vi "Create Initialize VIs.vi"   [LabVIEW 2015]
uses:
  Project Manipulation Scripts/Project Manipulation Scripts.lvlib
types:
  T1 = enum32{"invalid scope", "public", "private", "protected", "community"}
  T2 = enum32{"Invalid", "Standard", "Closed", "Hidden", "Minimized", "Maximized"}
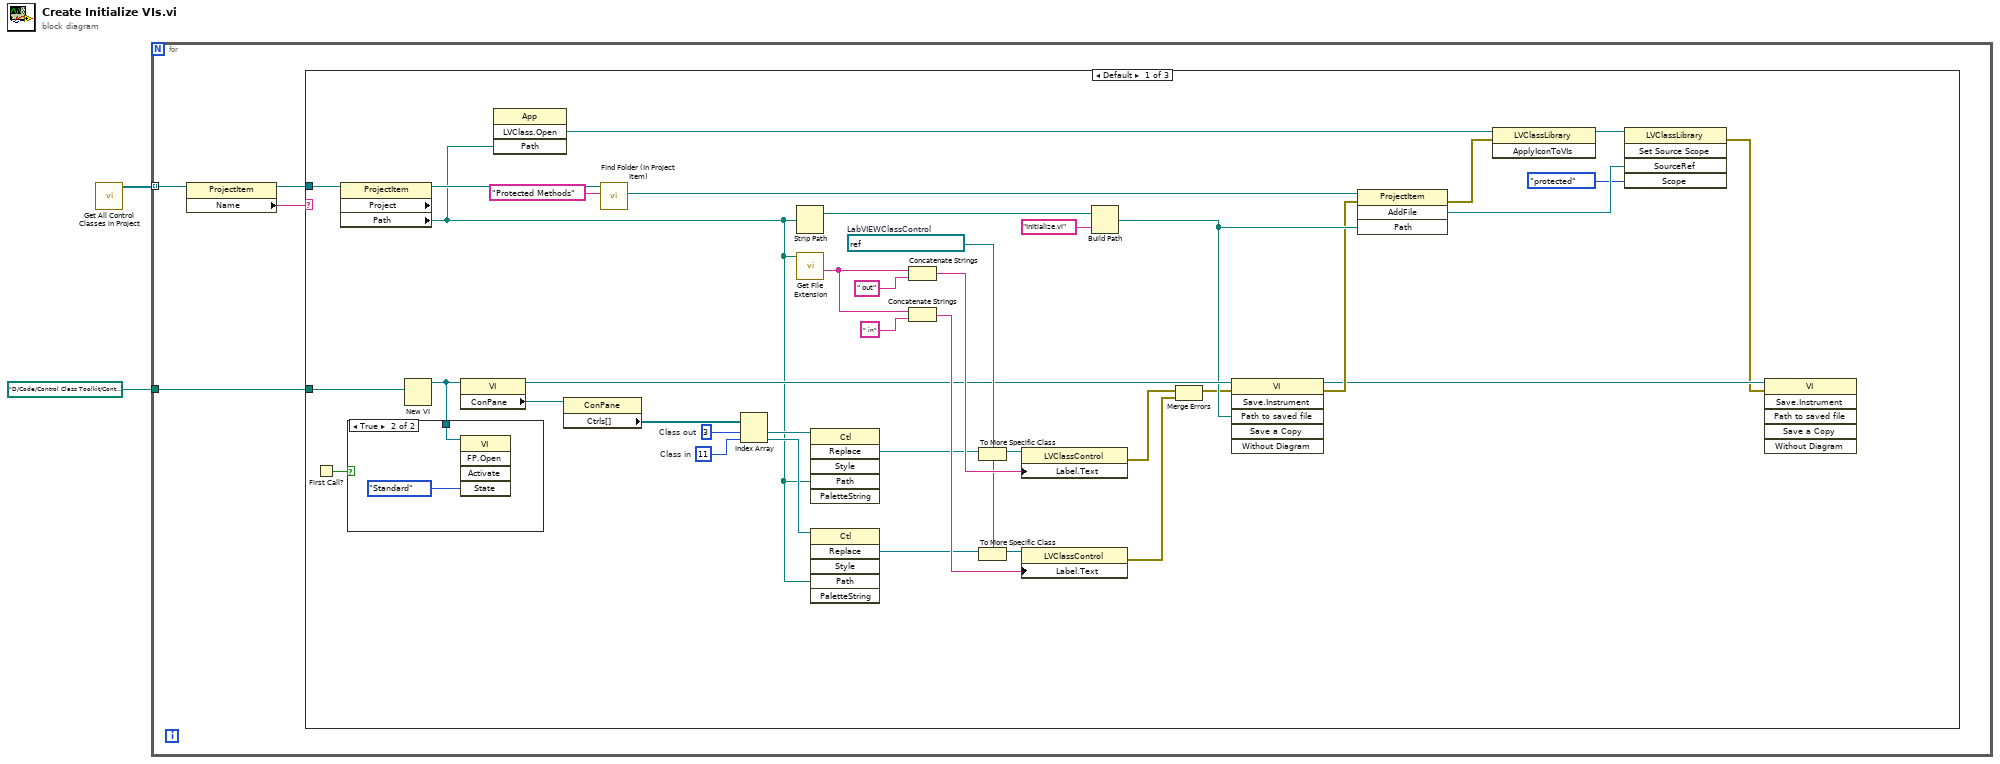
[diagram p0: block diagram]
diagram:
  n1 = call "Get All Control Classes in Project.vi"() -> ("All Control Classes"=w2:refnum<vi>[])  [unwired: 11 in]
  n2 = for {
    tunnel: w2 -> [w6] mode=indexing
    tunnel: path "D:/Code/Control Class Toolkit/Control Classes/Array/Initialize.vi" -> [w3]
    n3 = property class="ProjectItem"(reference=w6) -> (reference out=w4:refnum<vi>, "Name"=w5:string)  [unwired: 1 in, 1 out]
    n4 = case shown="Default" w5 {
      tunnel: w4 -> [w45 _ _]
      tunnel: w3 -> [w44 _ _]
      frame Default {
        w27 = refnum<vi> refnum  # LabVIEWClassControl
        w40 = 11  # Class in
        w41 = 3  # Class out
        n5 = First Call?() -> (First Call?: T/F=w7:bool)
        n6 = property class="ProjectItem" props=["Project", "Path"](reference=w45) -> (reference out=w22:refnum<vi>, "Path"=w15:path)  [unwired: 1 in, 2 out]
        n7 = New VI(10:w44) -> (3:w37:refnum<vi>)  [unwired: 6 in, 1 out]
        n8 = case shown="True" w7 {
          tunnel: w37 -> [_ w47]
          frame False {
          }
          frame True {
            n9 = invoke class="VI" method="FP.Open"(reference=w47, "State"=T2."Standard") -> ()  [unwired: 3 in, 5 out]
          }
        }
        n10 = property class="VI"(reference=w37) -> (reference out=w24:refnum<vi>, "ConPane"=w43:refnum<vi>)  [unwired: 1 in, 1 out]
        n11 = invoke class="App" method="LVClass.Open"("Path"=w15) -> ("LVClass.Open"=w14:refnum<vi>)  [unwired: 3 in, 3 out]
        n12 = property class="ConPane"(reference=w43) -> ("Ctrls[]"=w42:refnum<vi>[])  [unwired: 1 in, 2 out]
        n13 = call "Find Folder (In Project Item).vi"("Folder Name"="Protected Methods", "ProjectItem in"=w22) -> ("Folder Refnum"=w21:refnum<vi>)  [unwired: 7 in, 2 out]
        n14 = Index Array(array=w42, index #1=w41, index #2=w40) -> (element #1=w39:refnum<vi>, element #2=w38:refnum<vi>)
        n15 = Strip Path(path=w15) -> (stripped path=w26:path)  [unwired: 1 out]
        n16 = call <vilib>:"Get File Extension.vi"("file"=w15) -> ("filename without extension"=w34:string)  [unwired: 6 in, 4 out]
        n17 = invoke class="Ctl" method="Replace"(reference=w39, "Path"=w15) -> ("Replace"=w31:refnum<vi>)  [unwired: 4 in, 5 out]
        n18 = invoke class="Ctl" method="Replace"(reference=w38, "Path"=w15) -> ("Replace"=w29:refnum<vi>)  [unwired: 4 in, 5 out]
        n19 = Concatenate Strings(w34, " out" ("Label.Text")) -> (w33:string)
        n20 = Concatenate Strings(w34, " in" ("Label.Text")) -> (w32:string)
        n21 = To More Specific Class(target class=w27, reference=w31) -> (specific class reference=w30:refnum<vi>)  [unwired: 1 in, 1 out]
        n22 = To More Specific Class(target class=w27, reference=w29) -> (specific class reference=w28:refnum<vi>)  [unwired: 1 in, 1 out]
        n23 = property class="LVClassControl"(reference=w30, "Label.Text"=w33) -> (error out=w18:errorcluster)  [unwired: 1 in, 1 out]
        n24 = property class="LVClassControl"(reference=w28, "Label.Text"=w32) -> (error out=w17:errorcluster)  [unwired: 1 in, 1 out]
        n25 = Build Path(base path=w26, name or relative path="Initialize.vi") -> (appended path=w23:path)
        n26 = Merge Errors(w18, w17) -> (w16:errorcluster)
        n27 = invoke class="VI" method="Save.Instrument"(reference=w24, error in=w16, "Path to saved file"=w23) -> (reference out=w12:refnum<vi>, error out=w19:errorcluster)  [unwired: 3 in, 4 out]
        n28 = invoke class="ProjectItem" method="AddFile"(reference=w21, error in=w19, "Path"=w23) -> (error out=w13:errorcluster, "AddFile"=w10:refnum<vi>)  [unwired: 1 in, 2 out]
        n29 = invoke class="LVClassLibrary" method="ApplyIconToVIs"(reference=w14, error in=w13) -> (reference out=w11:refnum<vi>)  [unwired: 1 in, 2 out]
        n30 = invoke class="LVClassLibrary" method="Set Source Scope"(reference=w11, "SourceRef"=w10, "Scope"=T1."protected" ("scope")) -> (error out=w8:errorcluster)  [unwired: 2 in, 4 out]
        n31 = invoke class="VI" method="Save.Instrument"(reference=w12, error in=w8) -> ()  [unwired: 4 in, 6 out]
      }
      frame "Boolean.lvclass" {
      }
      frame "Array.lvclass", "Control.lvclass", "GObject.lvclass", "Generic.lvclass" {
      }
    }
  }
